vi "getSerializedData.vi"(0 "reference":refnum<class "StateTransitionEdge.lvclass">, 5 "error in (no error)":errorcluster) -> (14 "reference out":refnum<class "StateTransitionEdge.lvclass">, 15 "startNode":refnum<class "AbstractNode.lvclass">, 16 "endNode":refnum<class "AbstractNode.lvclass">, 17 "xmlOut":string, 19 "error out":errorcluster)   [LabVIEW 2014, in "StateTransitionEdge.lvclass"]
doc: "getSerializedData"
uses:
  <resource>/Framework/Providers/Open_GDS/UML/StateTransitionEdge_class/StateTransitionEdge.lvclass
  <resource>/Framework/Providers/Open_GDS/UML/AbstractNode_class/AbstractNode.lvclass
  <resource>/Framework/Providers/Open_GDS/UML/AbstractNode_class/ObjectReference.ctl
  <resource>/Framework/Providers/Open_GDS/UML/LineStyle_class/ObjectReference.ctl
  <resource>/Framework/Providers/Open_GDS/UML/ArrowHead_class/ObjectReference.ctl
  <resource>/Framework/Providers/Open_GDS/UML/General/Point/Point Point2D.ctl
  <resource>/Framework/Providers/Open_GDS/UML/BentStyle_class/ObjectReference.ctl
  <resource>/Framework/Providers/Open_GDS/UML/ReversedEngineering/ReversedEngineering_ViDependencyDetailsType.ctl
  <resource>/Framework/Providers/Open_GDS/UML/ArrowHead_class/ArrowHead.lvclass
  <resource>/Framework/Providers/Open_GDS/UML/BentStyle_class/BentStyle.lvclass
  <resource>/Framework/Providers/Open_GDS/UML/LineStyle_class/LineStyle.lvclass
  <resource>/Framework/Providers/Open_GDS/UML/ClassRelationshipEdge_class/ClassRelationshipEdge.lvclass
  <resource>/Framework/Providers/Open_GDS/UML/SegmentedLineEdge_class/SegmentedLineEdge.lvclass
  <resource>/Framework/Providers/Open_GDS/UML/AbstractEdge_class/AbstractEdge.lvclass
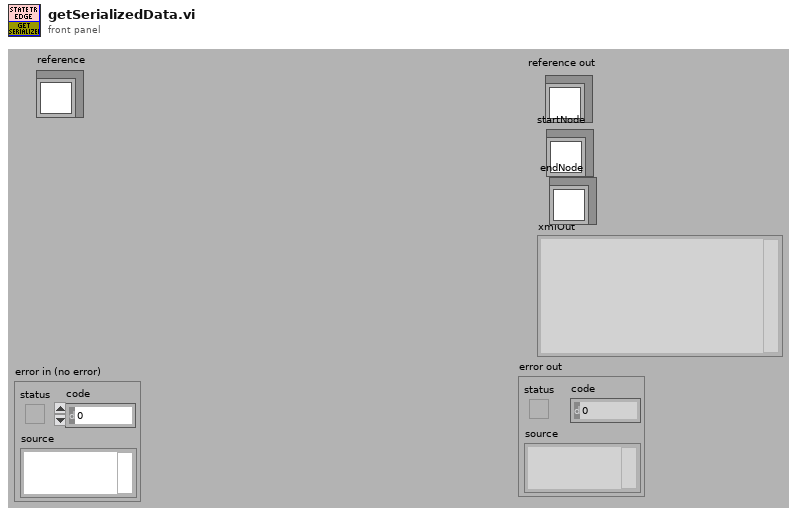
[diagram p1: front panel]
types:
  T1 = typedef "LineStyle.lvclass/ObjectReference.ctl" = refnum<k1>
  T2 = typedef "ArrowHead.lvclass/ObjectReference.ctl" = refnum<k1>
  T3 = typedef "Point Point2D.ctl" = cluster{"x":dbl, "y":dbl}
  T4 = typedef "BentStyle.lvclass/ObjectReference.ctl" = refnum<k1>
  T5 = typedef "ReversedEngineering_ViDependencyDetailsType.ctl" = cluster{"ThisVIs/Ctls":path[], "Dependent_VIs/Ctls":path[]}
  T6 = typedef "AbstractNode.lvclass/ObjectReference.ctl" = refnum<k1>
  T7 = cluster{"Base class":cluster{"Base class":cluster{"Base class":cluster{"Base class":cluster{"start":T6, "end":T6}}, "lineStyle":T1, "startArrowHead":T2, "endArrowHead":T2, "startLabel":string, "midLabel":string, "endLabel":string, "MidLabelOffset":T3, "SplitWire":bool}, "bentStyleRef":T4, "startConnectionOffset":cluster{"x":i32, "y":i32}, "endConnectionOffset":cluster{"x":i32, "y":i32}, "MidLineOffset":cluster{"x":i32, "y":i32}, "DepClass":T5}, "angle":dbl}
  T8 = typedef "StateTransitionEdge.lvclass/ObjectAttributes.ctl" = cluster{"angle":dbl}
  T9 = typedef "ClassRelationshipEdge.lvclass/ObjectAttributes.ctl" = cluster{"bentStyleRef":refnum<class "BentStyle.lvclass">, "startConnectionOffset":cluster{"x":i32, "y":i32}, "endConnectionOffset":cluster{"x":i32, "y":i32}, "MidLineOffset":cluster{"x":i32, "y":i32}, "DepClass":T5}
  T10 = typedef "SegmentedLineEdge.lvclass/ObjectAttributes.ctl" = cluster{"lineStyle":refnum<class "LineStyle.lvclass">, "startArrowHead":refnum<class "ArrowHead.lvclass">, "endArrowHead":refnum<class "ArrowHead.lvclass">, "startLabel":string, "midLabel":string, "endLabel":string, "MidLabelOffset":T3, "SplitWire":bool}
  T11 = typedef "AbstractEdge.lvclass/ObjectAttributes.ctl" = cluster{"start":refnum<class "AbstractNode.lvclass">, "end":refnum<class "AbstractNode.lvclass">}
  T12 = cluster{"Attributes":cluster{"Base class":cluster{"Base class":cluster{"Base class":cluster{"Base class":cluster{"start":T6, "end":T6}}, "lineStyle":T1, "startArrowHead":T2, "endArrowHead":T2, "startLabel":string, "midLabel":string, "endLabel":string, "MidLabelOffset":T3, "SplitWire":bool}, "bentStyleRef":T4, "startConnectionOffset":cluster{"x":i32, "y":i32}, "endConnectionOffset":cluster{"x":i32, "y":i32}, "MidLineOffset":cluster{"x":i32, "y":i32}, "DepClass":T5}, "angle":dbl}, "Type(String)":string, "Object name":string, "midLabel":string}
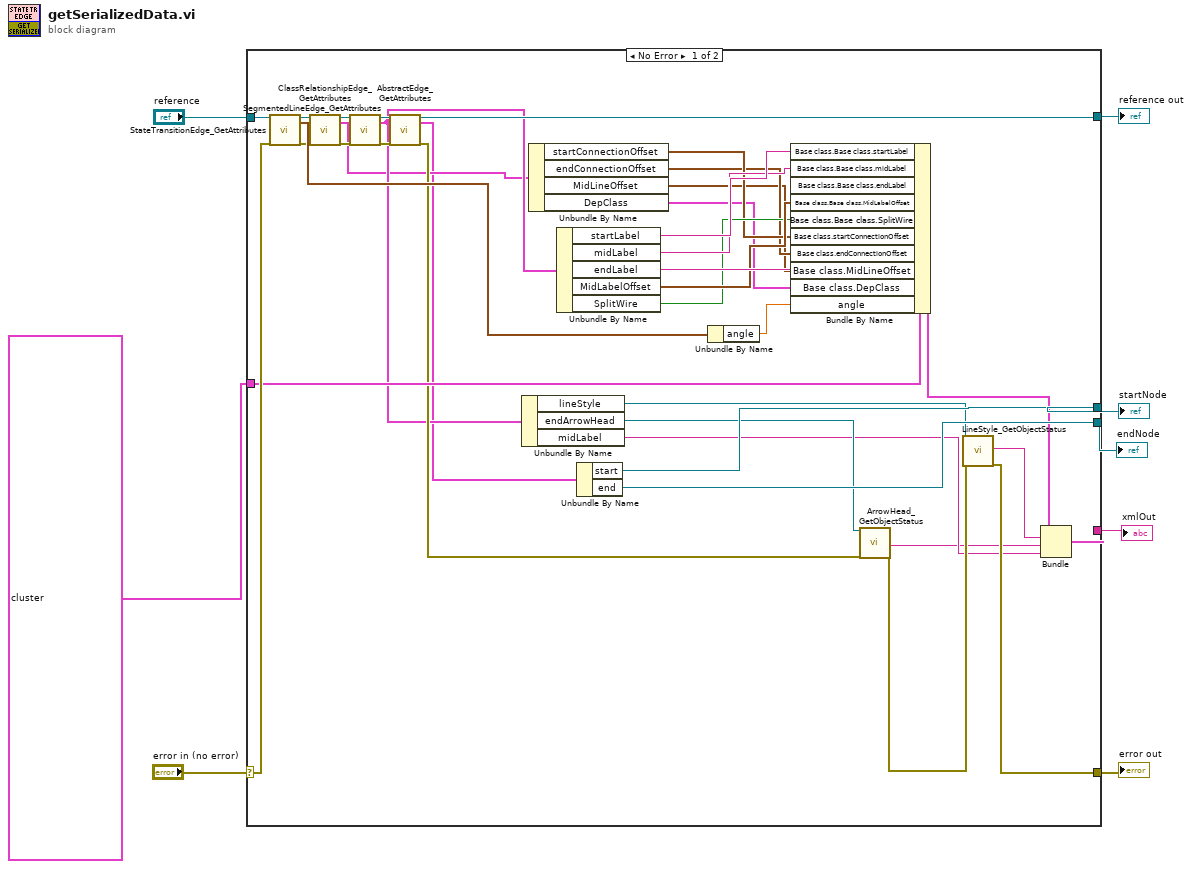
[diagram p0: block diagram]
diagram:
  n1 = case shown="No Error" "error in (no error)" {
    selector: "error in (no error)" -> [w45 w46]
    tunnel: "reference" -> [w44 w47]
    tunnel: [w37 w46] -> w6
    tunnel: [w14 w47] -> w5
    tunnel: [w42 _] -> w4
    tunnel: [w41 _] -> w3
    tunnel: [w40 _] -> w2
    tunnel: T7 {"Base class"={"Base class"={"Base class"={"Base class"={"start"=refnum, "end"=refnum}}, "lineStyle"=refnum, "startArrowHead"=refnum, "endArrowHead"=refnum, "startLabel"="", "midLabel"="", "endLabel"="", "MidLabelOffset"={"x"=0.0, "y"=0.0}, "SplitWire"=FALSE}, "bentStyleRef"=refnum, "startConnectionOffset"={"x"=0, "y"=0}, "endConnectionOffset"={"x"=0, "y"=0}, "MidLineOffset"={"x"=0, "y"=0}, "DepClass"={"ThisVIs/Ctls"=[], "Dependent_VIs/Ctls"=[]}}, "angle"=0.0} ("Attributes") -> [w34 _]
    frame No Error {
      n2 = call <resource>:"StateTransitionEdge_GetAttributes.vi"("reference in"=w44, "error in (no error)"=w45) -> ("reference out"=w21:refnum<class "StateTransitionEdge.lvclass">, "Data"=w22:T8, "error out"=w20:errorcluster)  [unwired: 1 in, 14 out]
      n3 = call <resource>:"ClassRelationshipEdge_GetAttributes.vi"("reference in"=w21, "error in (no error)"=w20) -> ("reference out"=w19:refnum<class "StateTransitionEdge.lvclass">, "Data"=w12:T9, "error out"=w18:errorcluster)  [unwired: 14 in, 1 out]
      n4 = call <resource>:"SegmentedLineEdge_GetAttributes.vi"("reference in"=w19, "error in (no error)"=w18) -> ("reference out"=w17:refnum<class "StateTransitionEdge.lvclass">, "Data"=w13:T10, "error out"=w16:errorcluster)  [unwired: 14 in, 1 out]
      n5 = call <resource>:"AbstractEdge_GetAttributes.vi"("reference in"=w17, "error in (no error)"=w16) -> ("reference out"=w14:refnum<class "StateTransitionEdge.lvclass">, "Data"=w11:T11, "error out"=w15:errorcluster)  [unwired: 14 in, 1 out]
      n6 = Unbundle By Name(w13) -> ("lineStyle"=w39:refnum<class "LineStyle.lvclass">, "endArrowHead"=w38:refnum<class "ArrowHead.lvclass">, "midLabel"=w35:string)
      n7 = Unbundle By Name(w12) -> ("startConnectionOffset"=w28:cluster{"x":i32, "y":i32}, "endConnectionOffset"=w27:cluster{"x":i32, "y":i32}, "MidLineOffset"=w26:cluster{"x":i32, "y":i32}, "DepClass"=w25:T5)
      n8 = Unbundle By Name(w13) -> ("startLabel"=w33:string, "midLabel"=w32:string, "endLabel"=w31:string, "MidLabelOffset"=w30:T3, "SplitWire"=w29:bool)
      n9 = Unbundle By Name(w11) -> ("start"=w41:refnum<class "AbstractNode.lvclass">, "end"=w40:refnum<class "AbstractNode.lvclass">)
      n10 = Unbundle By Name(w22) -> ("angle"=w24:dbl)
      n11 = Bundle By Name(cluster=w34, "Base class.Base class.startLabel"=w33, "Base class.Base class.midLabel"=w32, "Base class.Base class.endLabel"=w31, "Base class.Base class.MidLabelOffset"=w30, "Base class.Base class.SplitWire"=w29, "Base class.startConnectionOffset"=w28, "Base class.endConnectionOffset"=w27, "Base class.MidLineOffset"=w26, "Base class.DepClass"=w25, "angle"=w24) -> (w23:T7)
      n12 = call <resource>:"ArrowHead_GetObjectStatus.vi"("reference in"=w38, "error in (no error)"=w15) -> ("Object name"=w9:string, "error out"=w36:errorcluster)  [unwired: 1 in, 15 out]
      n13 = call <resource>:"LineStyle_GetObjectStatus.vi"("reference"=w39, "error in (no error)"=w36) -> ("Type(String)"=w10:string, "error out"=w37:errorcluster)  [unwired: 15 in, 1 out]
      n14 = Bundle("Attributes"=w23, "Type(String)"=w10, "Object name"=w9, "midLabel"=w35) -> (w43:T12)  [unwired: 1 out]
      n15 = Flatten To XML(anything=w43) -> (xml string=w42:string)
    }
    frame Error {
    }
  }
  "reference out" <- w5
  "error out" <- w6
  "startNode" <- w3
  "endNode" <- w2
  "xmlOut" <- w4
